vi "Read SubComponent Parameter - Raw.vi"(8 "error in (no error)":errorcluster, 10 "Parameter":string, 11 "Bus Monitor in":refnum<class "Bus Monitor.lvclass">) -> (0 "error out":errorcluster, 2 "Raw Data":u64 format="%016x")   [LabVIEW 2020, in "BCI-1553 API.lvlib" / "Bus Monitor.lvclass"]
doc: "<NO OPERATION ON BUS MONITOR>"
uses:
  Bus Monitor.lvclass
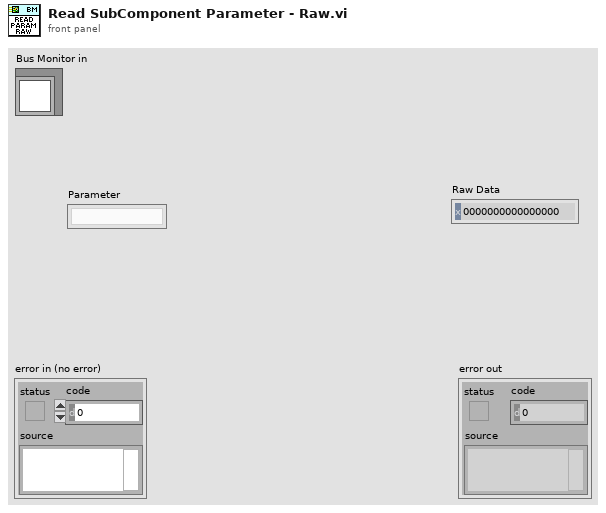
[diagram p1: front panel]
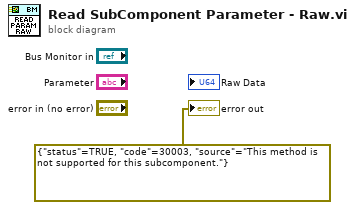
[diagram p0: block diagram]
diagram:
  "error out" <- errorcluster {"status"=TRUE, "code"=30003, "source"="This method is not supported for this subcomponent."} ("error out")
